vi "Obtain panel run registry DVR.vi"(8 "error in":errorcluster) -> (0 "error out":errorcluster, 3 "Panel registration DVR":refnum<data-value>)   [LabVIEW 2018, in "Fiber Auto Collimation References.lvclass"]
doc: "Creates or looks up a cross-library DVR used to keep track of all currently running panels. The DVR is for an array of Panel objects, each representing one currently running panel.\n\nNote: This does not track the Apex panel."
uses:
  Fiber Auto Collimation References.lvclass
  Panels/Fiber Auto Collimation panel.lvclass
  C:/Program Files (x86)/National Instruments/LabVIEW 2018/user.lib/nLight Tidbits/Cross-library references/Cross-library key/Cross-library key.lvclass
  409b8a44-1561-46b5-8a81-ab6b0300afa7.vi
  e253539d-0875-48cd-a2b7-b8d82f4e5496.vi
  409b8a44-1561-46b5-8a81-ab6b0300afa7.vi/b3628be3-34e6-46ff-84b6-fc4934738502.vi
  <userlib>/nLight Tidbits/Cross-library references/Cross-library key/Obtain cross library semaphore and acquire.vi
  409b8a44-1561-46b5-8a81-ab6b0300afa7.vi/83d6249a-ebc2-40b0-8445-304e2acc78f0.vi
  e253539d-0875-48cd-a2b7-b8d82f4e5496.vi/74008736-6506-49d3-aadf-455a30a88414.vi
  e253539d-0875-48cd-a2b7-b8d82f4e5496.vi/ac52ce72-1bf2-444f-96e9-87f43287f4cc.vi
  <userlib>/nLight Error Handling/Trash error.vi
  <vilib>/Utility/error.llb/Clear Errors.vi
  <vilib>/Utility/semaphor.llb/Obtain Semaphore Reference.vi
  <vilib>/Utility/semaphor.llb/Acquire Semaphore.vi
  <userlib>/nLight Error Handling/Log any errors.vi
  <userlib>/nLight Tidbits/Cross-library references/Cross-library key/Obtain class key.vi
  <vilib>/Utility/semaphor.llb/Release Semaphore.vi
  <vilib>/Utility/semaphor.llb/Release Semaphore Reference.vi
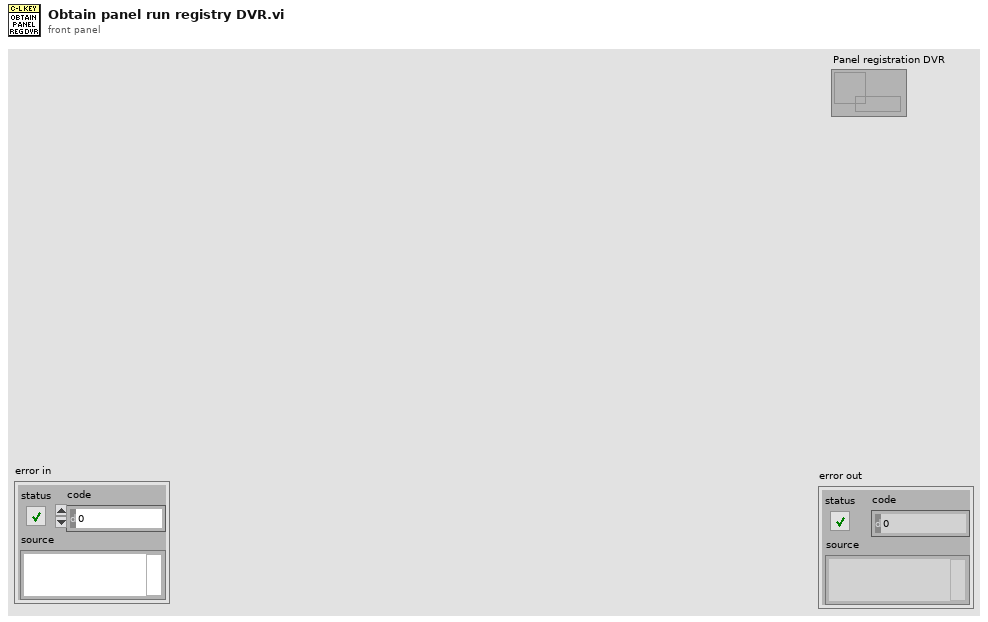
[diagram p1: front panel]
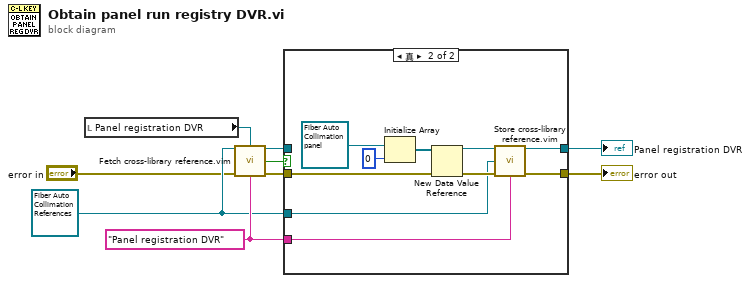
[diagram p0: block diagram]
diagram:
  w5 = refnum<class "Fiber Auto Collimation References.lvclass"> refnum ("nLight Station Template CLK.lvclass")
  w7 = "Panel registration DVR"
  n1 = local read "Panel registration DVR"() -> (w1:refnum<data-value>)
  n2 = call "Fetch cross-library reference.vim"("Cross-library key"=w5, "Reference type to fetch"=w1, "error in (no error)"="error in", "Specific ref type name [String/Enum]"=w7) -> ("Stored value (if present)"=w6:refnum<data-value>, "Nothing to fetch OR bad reference"=w9:bool, "error out"=w8:errorcluster)  [unwired: 9 in]
  n3 = case shown="真" w9 {
    tunnel: w8 -> [w11 w19]
    tunnel: w7 -> [_ w21]
    tunnel: [w11 w20] -> w3
    tunnel: w5 -> [_ w16]
    tunnel: [w10 w15] -> w4
    tunnel: w6 -> [w10 _]
    frame False {
    }
    frame True {
      n4 = Initialize Array(refnum<class "Fiber Auto Collimation panel.lvclass"> refnum ("Fiber Auto Collimation panel.lvclass"), 0 ("dimension size")) -> (w12:refnum<class "Fiber Auto Collimation panel.lvclass">[])
      n5 = New Data Value Reference(data value=w12, error in=w19) -> (data value reference=w18:refnum<data-value>, error out=w17:errorcluster)
      n6 = call "Store cross-library reference.vim"("Reference to store"=w18, "Cross-library key"=w16, "error in (no error)"=w17, "Specific ref type name [String/Enum]"=w21) -> ("Copy of stored reference"=w15:refnum<data-value>, "error out"=w20:errorcluster)  [unwired: 8 in, 2 out]
    }
  }
  "error out" <- w3
  "Panel registration DVR" <- w4
